vi "DAQmx Create Channel (AI-Acceleration-Accelerometer).vi"(0 "task in":refnum<k21>, 1 "maximum value":dbl=5.0 format="%0.2f", 2 "minimum value":dbl=-5.0 format="%0.2f", 3 "input terminal configuration":i32(ring)=-1 items=["default"=-1, "RSE"=10083, "NRSE"=10078, "Differential"=10106, "Pseudodifferential"=12529], 5 "physical channels":tag, 6 "current excitation source":i32(ring)=10200 items=["Internal"=10200, "External"=10167, "None"=10230], 7 "name to assign":string, 8 "current excitation value":dbl=0.004, 9 "units":i32(ring)=10186 items=["g"=10186, "m/s^2"=12470, "in/s^2"=12471, "From Custom Scale"=10065], 11 "error in":errorcluster, 12 "custom scale name":tag, 13 "sensitivity":dbl=1000.0, 14 "sensitivity units":i32(ring)=12509 items=["mVolts/g"=12509, "Volts/g"=12510]) -> (4 "task out":refnum<k21>, 15 "error out":errorcluster)   [LabVIEW 2020]
doc: "Creates channel(s) that use an accelerometer to measure acceleration."
uses:
  nilvaiu.dll
panel:
  # "input limits"
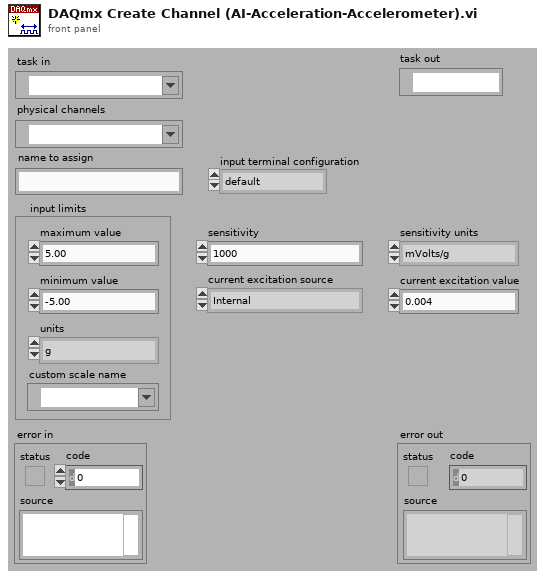
[diagram p1: front panel]
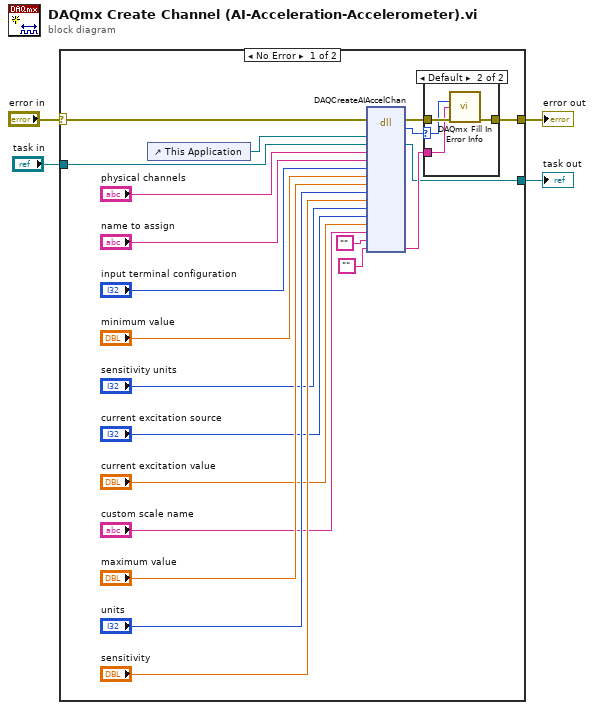
[diagram p0: block diagram]
diagram:
  n1 = case shown="No Error" "error in" {
    selector: "error in" -> [w17 w32]
    tunnel: [w18 w32] -> w2
    tunnel: "task in" -> [w19 w31]
    tunnel: [w20 w31] -> w1
    frame No Error {
      n2 = control-ref of="This Application"() -> (w22:refnum<vi>)
      n3 = dll-call lib="nilvaiu.*" fn="DAQCreateAIAccelChan"(error in=w17, "lvAppRef"=w22, "refObjPtr"=w19, "physicalChannelName"="physical channels", "channelNameIn"="name to assign", "terminalConfig"="input terminal configuration", "minVal"="minimum value", "maxVal"="maximum value", "units"="units", "sensitivity"="sensitivity", "sensitivityUnits"="sensitivity units", "currentExcitSrc"="current excitation source", "excitVal"="current excitation value", "customScaleName"="custom scale name", "channelNamesOut"="", "extendedErrorInfo"="") -> (error out=w25:errorcluster, "return type"=w24:i32, "refObjPtr"=w20:refnum<k21>, "extendedErrorInfo"=w23:string)  [unwired: 15 in, 1 out]
      n4 = case shown="Default" w24 {
        selector: w24 -> [_ w28]
        tunnel: w25 -> [w26 w30]
        tunnel: [w26 w29] -> w18
        tunnel: w23 -> [_ w27]
        frame 0 {
        }
        frame Default {
          n5 = call "DAQmx Fill In Error Info.vi"("status code"=w28, "extended error info"=w27, "error in"=w30) -> ("error out"=w29:errorcluster)  [unwired: 1 in, 11 out]
        }
      }
    }
    frame Error {
    }
  }
  "error out" <- w2
  "task out" <- w1
